vi "Configure IQ Skew Correction.vi"(8 "error in (no error)":errorcluster, 9 "Skew Path (0: RF)":u16(ring) items=["RF Output", "Baseband"], 10 "Enable Skew Correction (T:Enable)":bool=TRUE, 11 "VISA resource name":refnum<visa-resource-name>) -> (0 "error out":errorcluster, 3 "VISA resource name out":refnum<visa-resource-name>)   [LabVIEW 2011, in "Agilent PSG MXG Series.lvlib"]
doc: "Configures the I/Q skew correction function.\n\n<B>Notes:</B>\n(1) This VI is valid only in E8267C, E8267D.\n\n(2) For E8267C, this VI is valid only when the instrument installs <B>Option 002</B> (Internal baseband generator) or <B>Option 602</B> (Digital bus baseband generator)."
uses:
  Agilent PSG MXG Series.lvlib
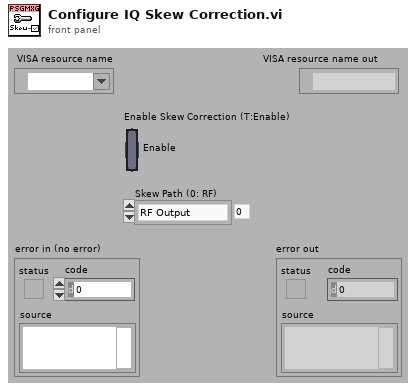
[diagram p1: front panel]
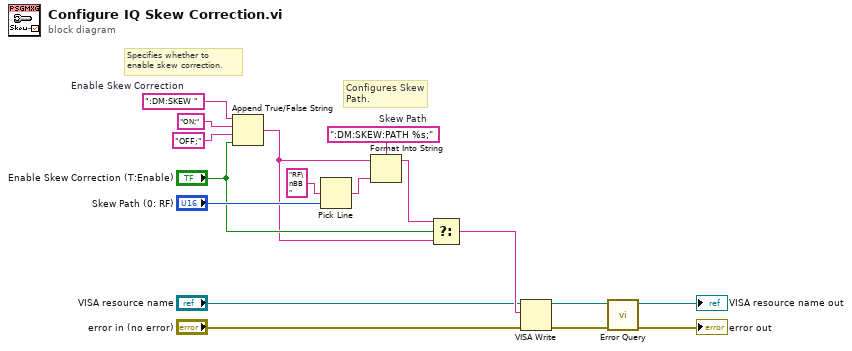
[diagram p0: block diagram]
diagram:
  w14 = ":DM:SKEW:PATH %s;"  # Skew Path
  w17 = ":DM:SKEW "  # Enable Skew Correction
  # "Configures Skew\nPath."
  # "Specifies whether to\nenable skew correction."
  n1 = Append True/False String(1:"Enable Skew Correction (T:Enable)", 2:"OFF;" ("false string"), 3:"ON;" ("true string"), 4:w17) -> (0:w8:string)
  n2 = Pick Line(multi-line string="RF\nBB", line index="Skew Path (0: RF)") -> (output string=w13:string)  [unwired: 1 in]
  n3 = Format Into String(format string=w14, initial string=w8, w13) -> (resulting string=w9:string)  [unwired: 1 in, 1 out]
  n4 = Select(t=w9, s="Enable Skew Correction (T:Enable)", f=w8) -> (s? t:f=w5:string)
  n5 = VISA Write(VISA resource name="VISA resource name", write buffer=w5, error in (no error)="error in (no error)") -> (VISA resource name out=w7:refnum<visa-resource-name>, error out=w6:errorcluster)  [unwired: 1 out]
  n6 = call "Error Query.vi"("error in (no error)"=w6, "VISA resource name"=w7) -> ("error out"=→"error out":errorcluster, "VISA resource name out"=→"VISA resource name out":refnum<visa-resource-name>)  [unwired: 6 in, 2 out]
